vi "singleEvent.vi"(8 "Event":string, 9 "View":string, 10 "Debug":bool, 11 "httpRequestID":u32) -> ()   [LabVIEW 2014]
uses:
  FRCts20_EspEngine.lvlib
  <vilib>/wsapi/NI_WebServices.lvlib
  <vilib>/wsapi/subVIs/Set Boolean ESP Variable.vi
  Web Methods/source/VI Source/Web Method Public Interface/FRCts20_WebMethods_ctl_teamIdentifier.ctl
  Web Methods/source/VI Source/FRCts20_WebMethods.lvlib
  Web Methods/source/VI Source/Web Method Public Interface/FRCts20_WebMethods_ctl_singleEvent.ctl
panel:
  in  "Single Event":T1={"Team"=[{"Team Nickname"="One", "Team Number "=11, "UniqueId"=1}, {"Team Nickname"="Two", "Team Number "=22, "UniqueId"=2}, {"Team Nickname"="Three", "Team Number "=33, "UniqueId"=3}], "Issue Count"=0, "Location"="New York City", "Start Date "=timestamp(0 s since 1904-01-01)}
  out "error out":errorcluster
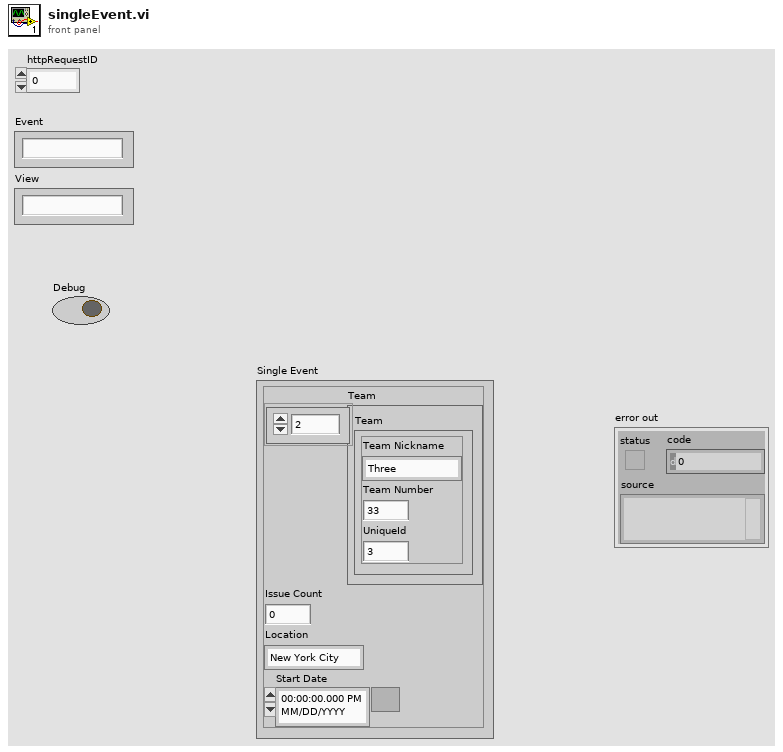
[diagram p1: front panel]
types:
  T1 = typedef "FRCts20_WebMethods.lvlib/FRCts20_WebMethods_ctl_singleEvent.ctl" = cluster{"Team":T2[], "Issue Count":i32, "Location":string, "Start Date ":timestamp}
  T2 = typedef "FRCts20_WebMethods.lvlib/FRCts20_WebMethods_ctl_teamIdentifier.ctl" = cluster{"Team Nickname":string, "Team Number ":u32, "UniqueId":u32}
  T3 = typedef "FRCts20_EspEngine.lvlib/FRCts20_EspEngine_SearchBrowser.ctl" = cluster{"Event":cluster{"Event Index":u32, "Event Name":string, "Start Time":timestamp, "End Time":timestamp, "OpenIssues":u8, "IsLive":bool}[], "select-choice-software":string, "select-choice-location":string}
  T4 = typedef "FRCts20_EspEngine.lvlib/FRCts20_EspEngine_Event.ctl" = cluster{"Single Event":T1, "EventOpenIssueCount":i16, "Requests":cluster{"RequestId":i32, "Request Description":string, "Team Number":i32}[], "ClosedRequests":cluster{"RequestId":i32, "Request Description":string, "Team Number":i32}[], "NotFoundStatus":bool}
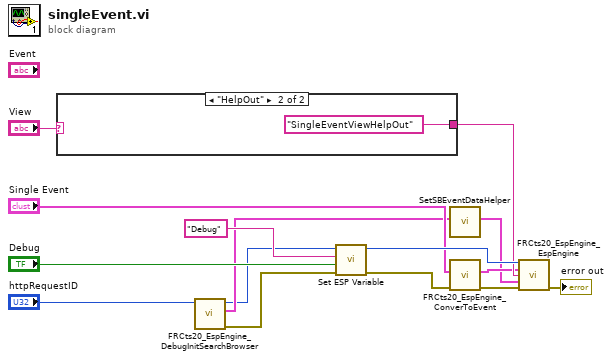
[diagram p0: block diagram]
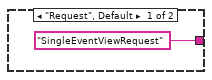
[diagram p2: hidden frame]
diagram:
  n1 = case shown="\"HelpOut\"" "View" {
    tunnel: ["SingleEventViewRequest" "SingleEventViewHelpOut"] -> w7
    frame "Request", Default {
    }
    frame "HelpOut" {
    }
  }
  n2 = call "FRCts20_EspEngine_DebugInitSearchBrowser.vi"("httpRequestID"="httpRequestID") -> ("error out"=w3:errorcluster, "SearchBrowser"=w5:T3, "httpRequestID out"=w1:u32)  [unwired: 8 in]
  n3 = call-poly <vilib>:"Set ESP Variable.vi"("error in (no error)"=w3, "value"="Debug", "key"="Debug", "httpRequestID"=w1) -> ("error out"=w9:errorcluster, "httpRequestID out"=w13:u32)  [unwired: 6 in]
  n4 = call "SetSBEventDataHelper.vi"("SearchBrowser"=w5) -> ("SearchBrowser"=w4:T3)  [unwired: 10 in]
  n5 = call "FRCts20_EspEngine_ConverToEvent.vi"("error in (no error)"=w9, "Single Event"="Single Event") -> ("error out"=w8:errorcluster, "Event"=w6:T4)  [unwired: 8 in]
  n6 = call "FRCts20_EspEngine_EspEngine.vi"("httpRequestID"=w13, "Cluster"=w6, "Page"=w7, "SearchBrowser"=w4, "error in (no error)"=w8) -> ("error out"=→"error out":errorcluster)  [unwired: 9 in, 1 out]
